vi "GetFGenBdcstEvents.vi"() -> (3 "Event Registration Refnum":refnum<event-registration>)   [LabVIEW 2018, in "Test.lvclass"]
uses:
  Test.lvclass
  FGen/FgenModule/Protected/clEventType.ctl
  FGen/FgenModule/FgenModule.lvlib
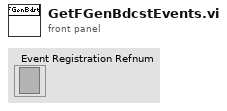
[diagram p1: front panel]
types:
  T1 = typedef "FgenModule.lvlib/clBroadcastEvents.ctl" = cluster{"DidInit":refnum<user-event>, "StatusUpdate":refnum<user-event>, "ErrorReport":refnum<user-event>, "DidStop":refnum<user-event>, "PathToINI":refnum<user-event>, "Channels":refnum<user-event>, "Function":refnum<user-event>, "Waveforms":refnum<user-event>, "Triggers":refnum<user-event>, "FunctionParams":refnum<user-event>, "FunctionArbs":refnum<user-event>, "FunctionSampleRate":refnum<user-event>}
  T2 = cluster{"FunctionSampleRate":refnum<user-event>, "FunctionArbs":refnum<user-event>, "FunctionParams":refnum<user-event>, "Function":refnum<user-event>, "ErrorReport":refnum<user-event>}
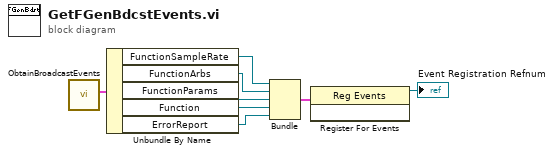
[diagram p0: block diagram]
diagram:
  n1 = call "ObtainBroadcastEvents.vi"() -> ("clBroadcastEvents"=w8:T1)  [unwired: 10 in, 1 out]
  n2 = Unbundle By Name(w8) -> ("FunctionSampleRate"=w2:refnum<user-event>, "FunctionArbs"=w3:refnum<user-event>, "FunctionParams"=w4:refnum<user-event>, "Function"=w7:refnum<user-event>, "ErrorReport"=w5:refnum<user-event>)
  n3 = Bundle("FunctionSampleRate"=w2, "FunctionArbs"=w3, "FunctionParams"=w4, "Function"=w7, "ErrorReport"=w5) -> (w6:T2)  [unwired: 1 in]
  n4 = register-events(w6) -> (reference out=→"Event Registration Refnum":refnum<event-registration>)  [unwired: 2 in, 1 out]
